vi "EF_CalcTimeTrace.vi"(7 "DeltaT":dbl caption="dt / ms:" format="%.2f", 9 "TimeTrace":u32[](array[numeric]), 10 "Bin":i32, 11 "Total bin":u64) -> (0 "TimeTrace_out":u32[](array[numeric]), 1 "dt":dbl, 2 "T0":dbl)   [LabVIEW 2017]
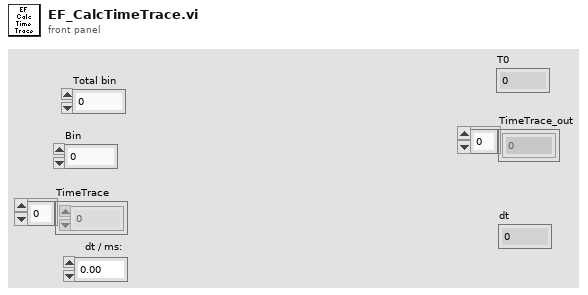
[diagram p1: front panel]
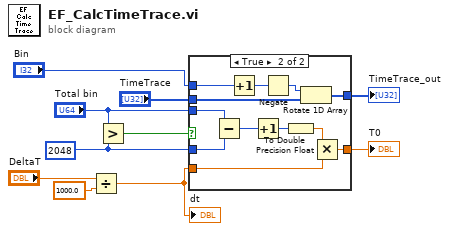
[diagram p0: block diagram]
diagram:
  w1 = u64 2048 ("y")
  n1 = Divide(x="DeltaT", y=1000.0) -> (x/y=w2:dbl)
  "dt" <- w2
  n2 = Greater?(x="Total bin", y=w1) -> (0:w9:bool)
  n3 = case shown="True" w9 {
    tunnel: "Total bin" -> [_ w15]
    tunnel: w2 -> [_ w23]
    tunnel: [_ w22] -> w10
    tunnel: "Bin" -> [_ w17]
    tunnel: "TimeTrace" -> [w11 w19]
    tunnel: [w11 w18] -> w6
    tunnel: w1 -> [_ w12]
    frame False {
    }
    frame True {
      n4 = Subtract(x=w15, y=w12) -> (x-y=w14:u64)
      n5 = Increment(x=w17) -> (x+1=w20:i32)
      n6 = Increment(x=w14) -> (x+1=w13:u64)
      n7 = Negate(x=w20) -> (-x=w21:i32)
      n8 = To Double Precision Float(number=w13) -> (double precision float=w16:dbl)
      n9 = Rotate 1D Array(1:w19, 2:w21) -> (0:w18:u32[])
      n10 = Multiply(x=w16, y=w23) -> (x*y=w22:dbl)
    }
  }
  "TimeTrace_out" <- w6
  "T0" <- w10
